vi "SS GUI Measurement setup.vi"(9 "SS measurement":T1={"Signal frequencies (Hz)"=[1000.0], "Signal amplitudes (V)"=[0.707], "Sampling frequencies (Hz)"=[10000000.0], "Record lengths (multiples of periods)"=[10000.0], "Calculate results"=FALSE, "Algorithm"="TWM-WFFT", "TWM data directories"=[], "TWM data directories relative"=[], "Settle down after AC source change (s)"=1.0, "PJVS frequencies (Hz)"=[1000.0], "PJVS reference voltages array of vector cluster"=[{"PJVS reference voltages vector"=[]}], "Requested PJVS steps"=[20], "Measure CE"=FALSE, "Measure CE before"=FALSE, "Measure CE after"=FALSE, "Single point CE measurement"=FALSE, "original CE template path"=path "", "new CE template path before SS"=path "", "new CE template path before SS relative"=path "", "new CE template path after SS"=path "", "new CE template path after SS relative"=path "", "original CE fit path"=path "", "new CE fit path before SS"=path "", "new CE fit path before SS relative"=path "", "new CE fit path after SS"=path "", "new CE fit path after SS relative"=path "", "Measure digitizer gain"=FALSE, "Measure digitizer gain before"=FALSE, "Measure digitizer gain after"=FALSE, "Digitizer gain"=0.0, "Data folder"=path "", "FR fit path"=path "", "new FR fit path relative"=path "", "Rs"=0, "Re"=0, "SS measurement info files"=[]} {"PJVS reference voltages array of vector cluster"."PJVS reference voltages vector" format="%#_3p"; "PJVS frequencies (Hz)" format="%#_3p"; "Record lengths (multiples of periods)" format="%#_3p"; "Sampling frequencies (Hz)" format="%#_3p"; "Signal amplitudes (V)" format="%#_3p"; "Signal frequencies (Hz)" format="%#_3p"}) -> (3 "SS measurement out":T1={"Signal frequencies (Hz)"=[1000.0], "Signal amplitudes (V)"=[0.707], "Sampling frequencies (Hz)"=[10000000.0], "Record lengths (multiples of periods)"=[10000.0], "Calculate results"=FALSE, "Algorithm"="TWM-WFFT", "TWM data directories"=[], "TWM data directories relative"=[], "Settle down after AC source change (s)"=1.0, "PJVS frequencies (Hz)"=[1000.0], "PJVS reference voltages array of vector cluster"=[{"PJVS reference voltages vector"=[]}], "Requested PJVS steps"=[20], "Measure CE"=FALSE, "Measure CE before"=FALSE, "Measure CE after"=FALSE, "Single point CE measurement"=FALSE, "original CE template path"=path "", "new CE template path before SS"=path "", "new CE template path before SS relative"=path "", "new CE template path after SS"=path "", "new CE template path after SS relative"=path "", "original CE fit path"=path "", "new CE fit path before SS"=path "", "new CE fit path before SS relative"=path "", "new CE fit path after SS"=path "", "new CE fit path after SS relative"=path "", "Measure digitizer gain"=FALSE, "Measure digitizer gain before"=FALSE, "Measure digitizer gain after"=FALSE, "Digitizer gain"=0.0, "Data folder"=path "", "FR fit path"=path "", "new FR fit path relative"=path "", "Rs"=0, "Re"=0, "SS measurement info files"=[]} {"PJVS reference voltages array of vector cluster"."PJVS reference voltages vector" format="%#_3p"; "PJVS frequencies (Hz)" format="%#_3p"; "Record lengths (multiples of periods)" format="%#_3p"; "Sampling frequencies (Hz)" format="%#_3p"; "Signal amplitudes (V)" format="%#_3p"; "Signal frequencies (Hz)" format="%#_3p"})   [LabVIEW 2020]
uses:
  SS Measurement/Type definitions/SS measurement.ctl
  <vilib>/Utility/error.llb/Error Cluster From Error Code.vi
  <vilib>/ErrorRing/Error Ring.xnode
  external libraries/varilib/varilib.lvlib
panel:
  in  "TabCEmeas":enum32{"Measure CE", "Without CE meas."}(tab)
  in  "Measure CE before":bool caption="before"
  in  "Measure CE after":bool caption="after"
  in  "RadioCEmeastype":enum32{"single point", "template"}(radio) caption="Method:"
  in  "orignal CE template path":path caption="CE template path:"
  in  "original CE fit path":path caption="Use file with CE fit:"
  in  "Re":i32 min=0 step=1
  in  "Rs":i32 min=0 step=1
  out "PJVS triangles error":string="!"
  out "PJVS triangles in record":dbl
  out "No of samples":dbl format="%#_6p"
  out "Sampling time (s)":dbl
  in  "original FR fit path":path caption="FR fit path:"
  out "DG error":string="!"
  in  "RadioGain":enum32{"DGmeasure", "DGvalue"}(radio)
  in  "Measure gain after":bool caption="after"
  in  "Measure gain before":bool caption="before"
  in  "Digitizer gain":dbl=1.0 min=1e-07 max=10000000000.0 format="%_7g"
  out "Is coherent":string="!"
  out "CE error":string="!"
  in  "Data folder":path caption="Save data to folder:"
  in  "Requested PJVS steps":u32
  out "Requested PJVS steps out":u32[](array[numeric])
  in  "PJVS frequency (Hz)":dbl
  out "PJVS frequencies (Hz) out":dbl[](array[numeric])
  in  "Record length (multiple of period)":dbl
  in  "Signal frequency (Hz)":dbl format="%#_7p"
  in  "Calculate results":bool
  in  "Algorithm":string
  out "Signal amplitudes (V) out":dbl[](array[numeric])
  out "Record lengths (multiples of period)":dbl[](array[numeric])
  out "Sampling frequencies (Hz) out":dbl[](array[numeric])
  out "Signal frequencies out (Hz)":dbl[](array[numeric]) caption="List of measurement frequencies" format="%#_7p"
  in  "Settle down after AC\nsource change (s)":dbl=1.0 format="%#_13g"
  in  "Sampling frequency (Hz)":dbl=10000000.0 format="%#_13p"
  in  "Signal amplitude (V)":dbl=1.0 format="%#_13g"
  in  "show connections":bool
  out "gui_elements":refnum<vi>[](array[refnum])
  in  "save_and_quit":bool
  in  "cancel":bool
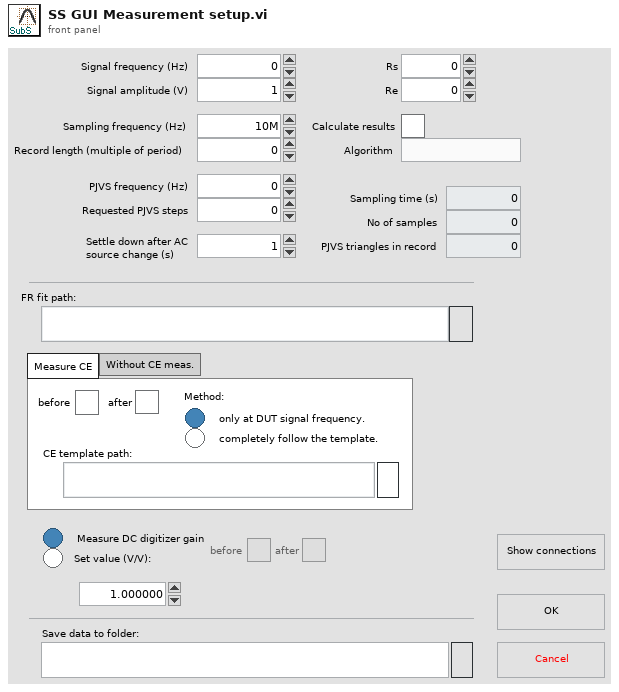
[diagram p1: front panel]
types:
  T1 = typedef "SS measurement.ctl" = cluster{"Signal frequencies (Hz)":dbl[], "Signal amplitudes (V)":dbl[], "Sampling frequencies (Hz)":dbl[], "Record lengths (multiples of periods)":dbl[], "Calculate results":bool, "Algorithm":string, "TWM data directories":path[], "TWM data directories relative":path[], "Settle down after AC source change (s)":dbl, "PJVS frequencies (Hz)":dbl[], "PJVS reference voltages array of vector cluster":cluster{"PJVS reference voltages vector":dbl[]}[], "Requested PJVS steps":u32[], "Measure CE":bool, "Measure CE before":bool, "Measure CE after":bool, "Single point CE measurement":bool, "original CE template path":path, "new CE template path before SS":path, "new CE template path before SS relative":path, "new CE template path after SS":path, "new CE template path after SS relative":path, "original CE fit path":path, "new CE fit path before SS":path, "new CE fit path before SS relative":path, "new CE fit path after SS":path, "new CE fit path after SS relative":path, "Measure digitizer gain":bool, "Measure digitizer gain before":bool, "Measure digitizer gain after":bool, "Digitizer gain":dbl, "Data folder":path, "FR fit path":path, "new FR fit path relative":path, "Rs":i32, "Re":i32, "SS measurement info files":path[]}
  T2 = enum32{"Bad", "Idle", "Run top level", "Running"}
  T3 = cluster{"PJVS reference voltages vector":dbl[]}[]
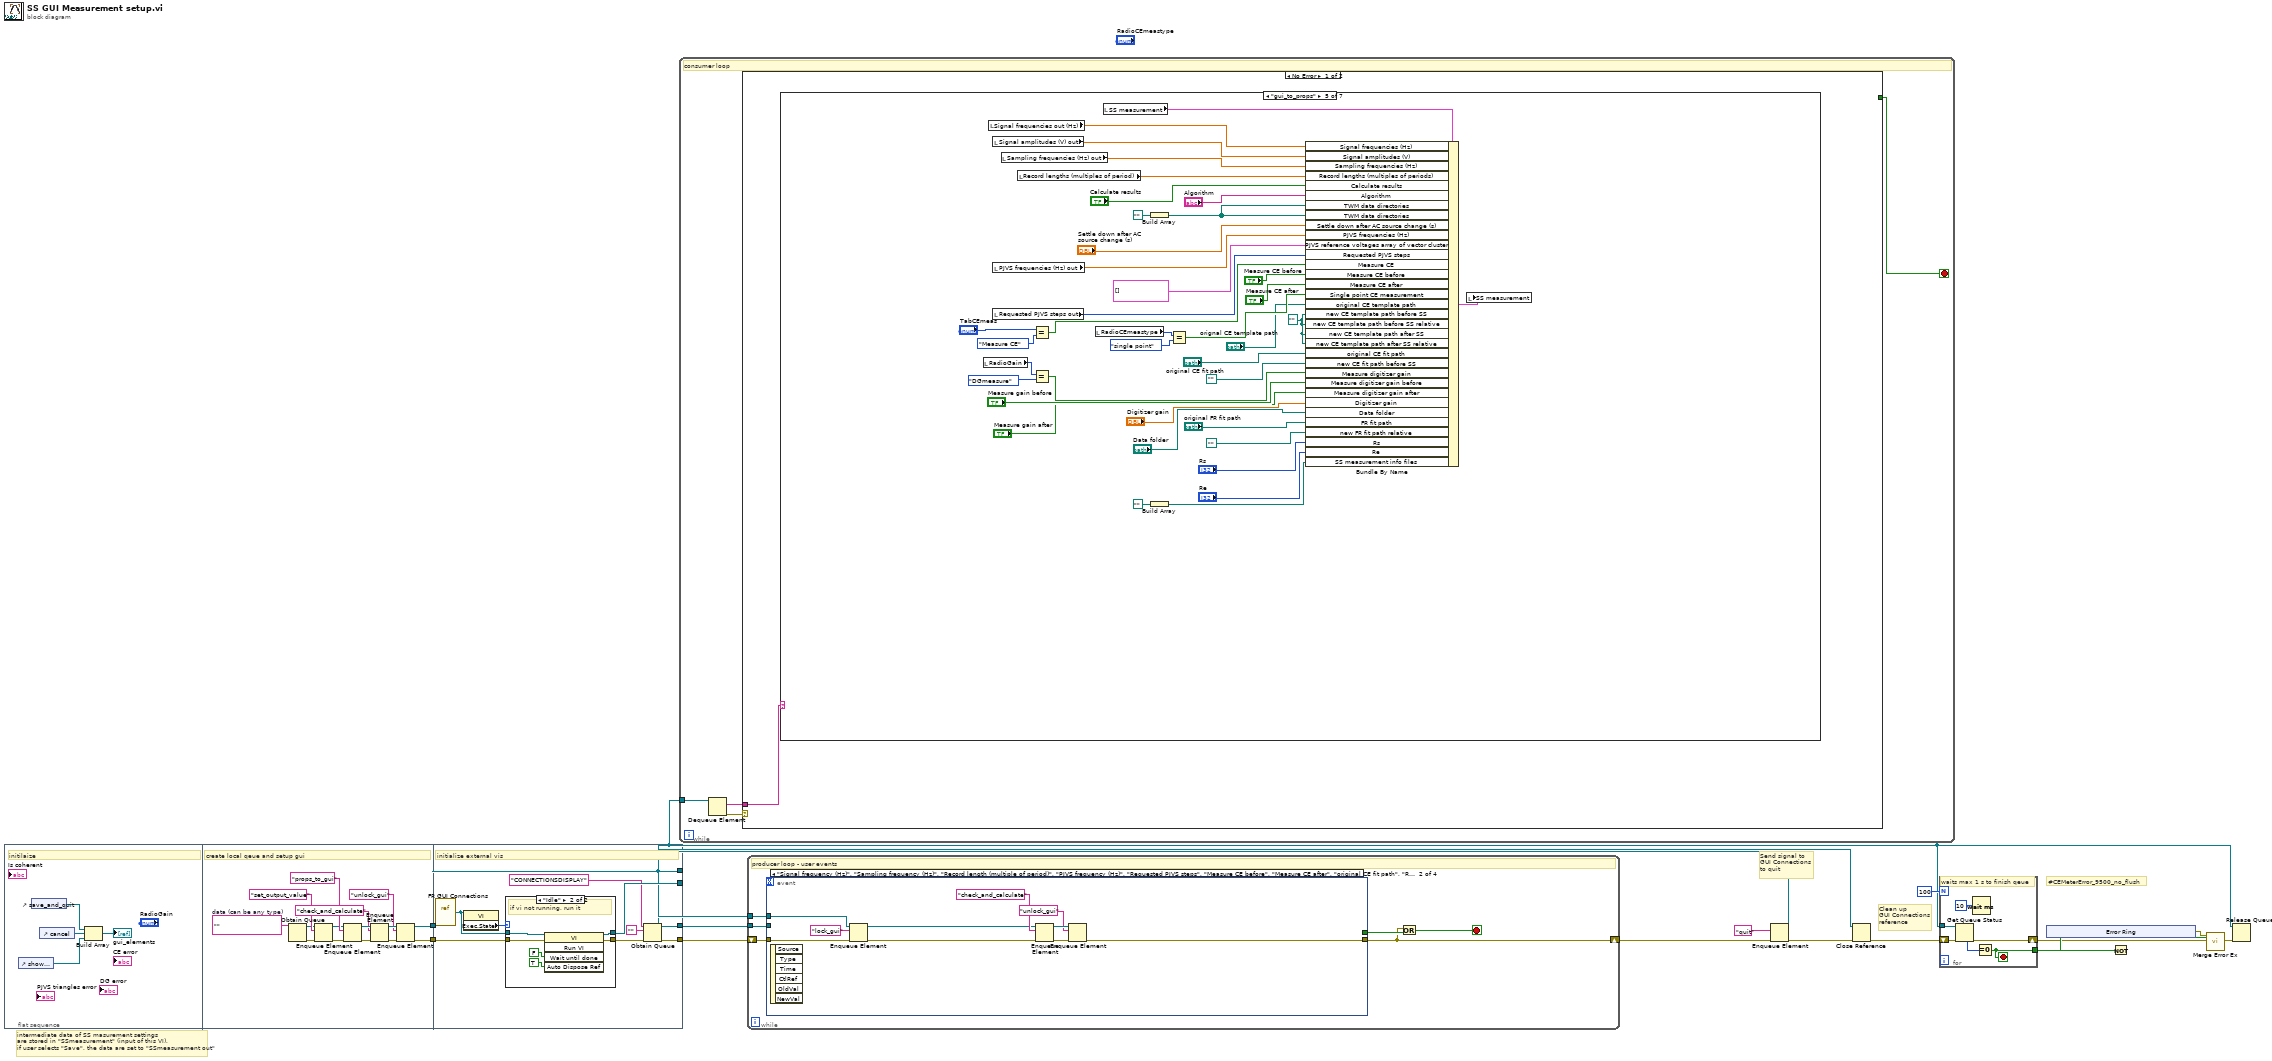
[diagram p0: block diagram]
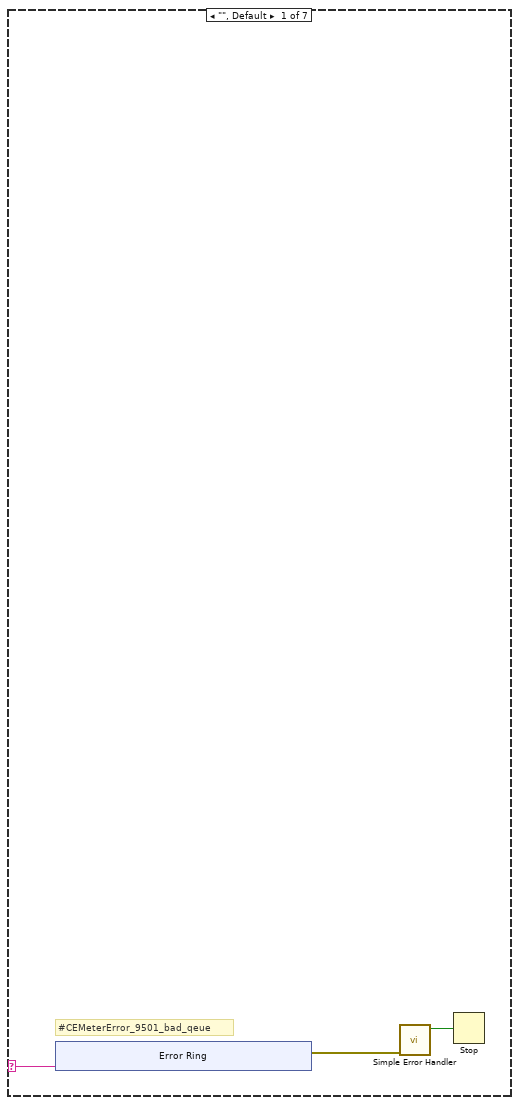
[diagram p3: hidden frame]
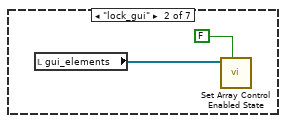
[diagram p4: hidden frame]
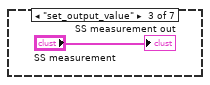
[diagram p5: hidden frame]
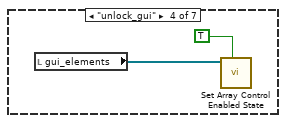
[diagram p6: hidden frame]
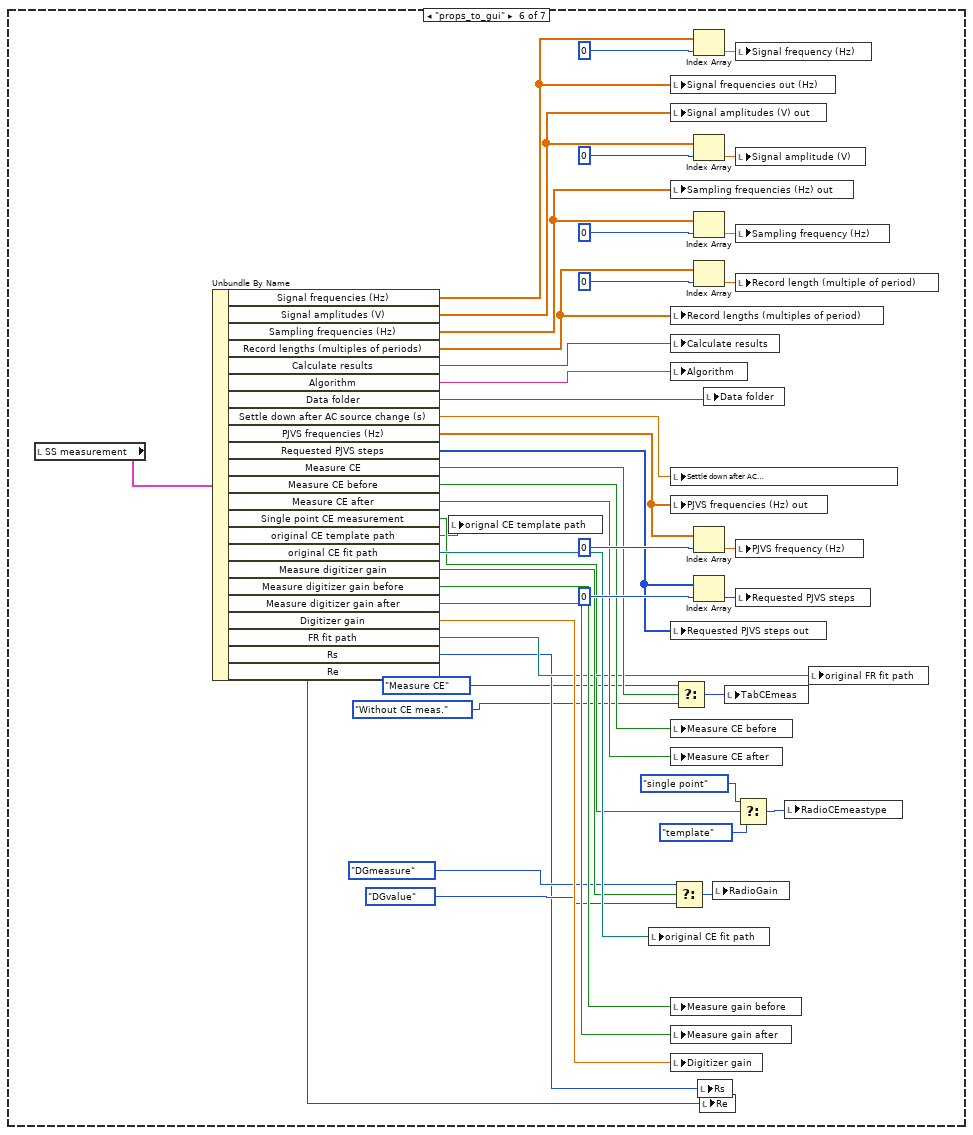
[diagram p7: hidden frame]
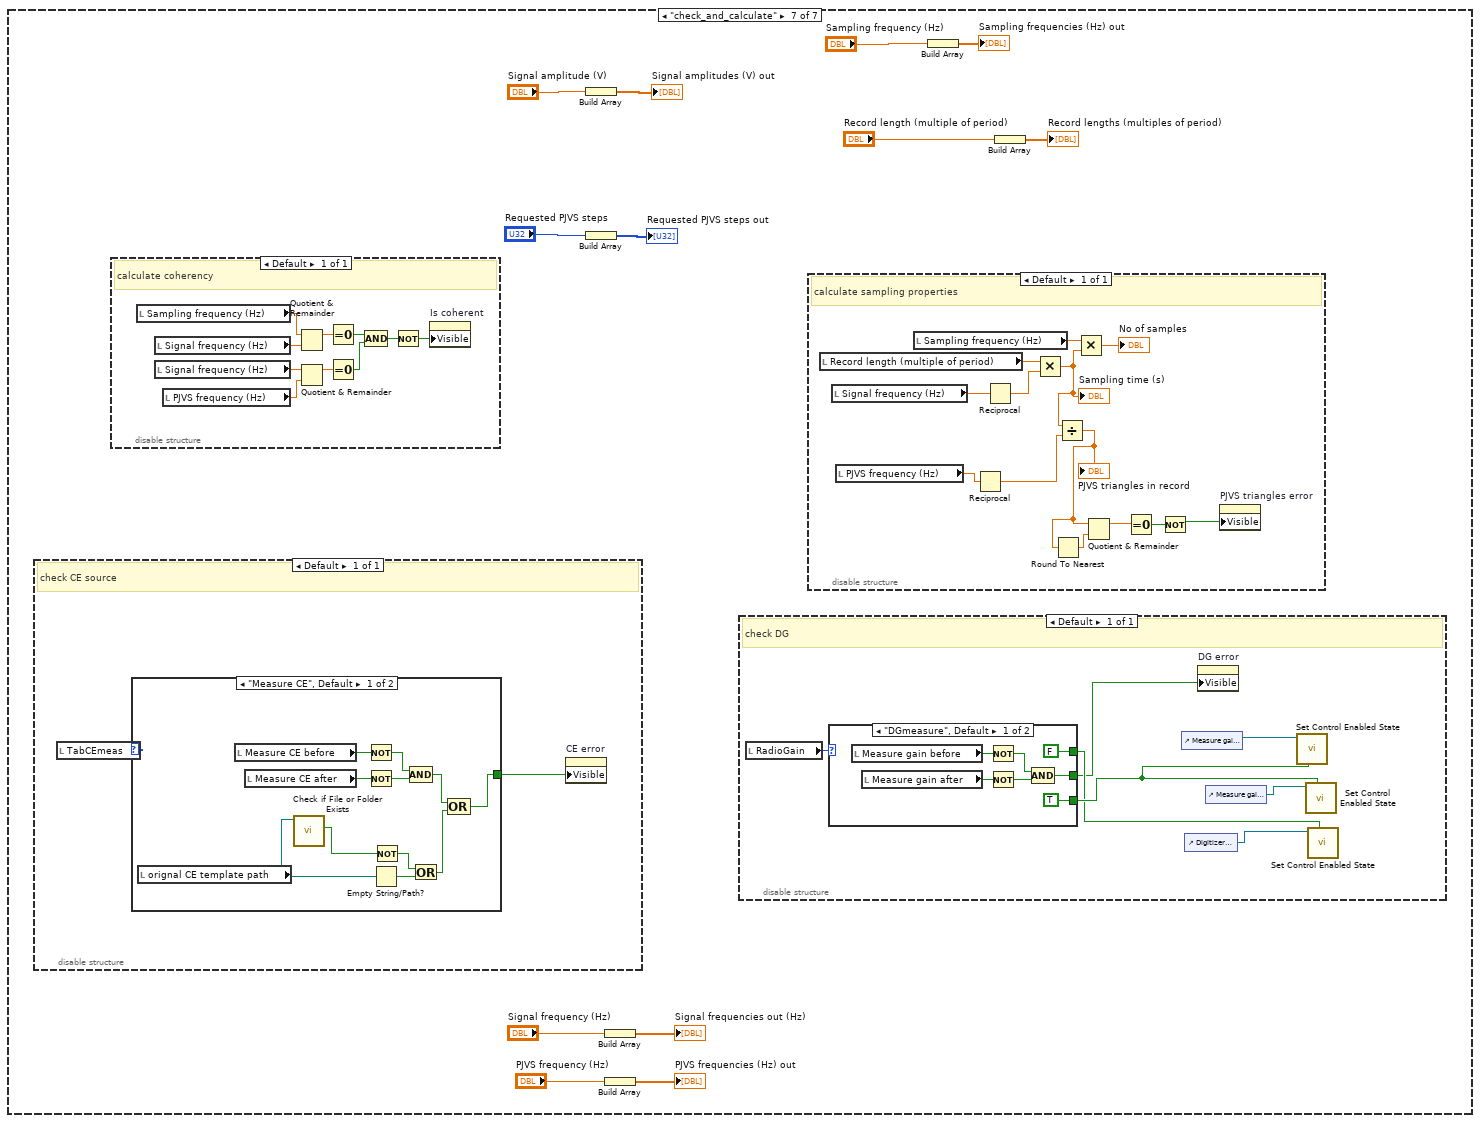
[diagram p8: hidden frame]
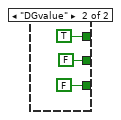
[diagram p9: hidden frame]
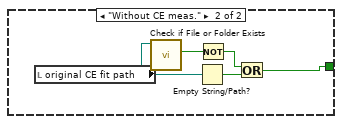
[diagram p10: hidden frame]
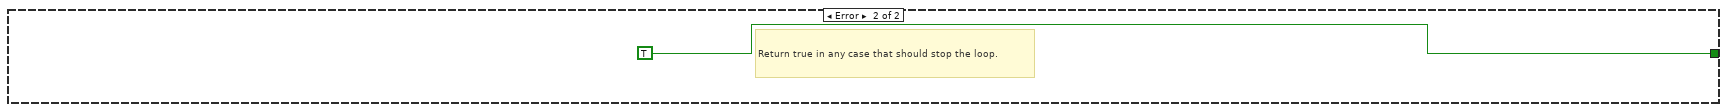
[diagram p11: hidden frame]
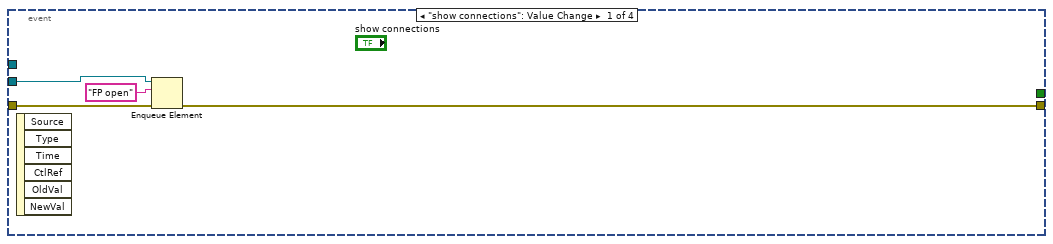
[diagram p12: hidden frame]
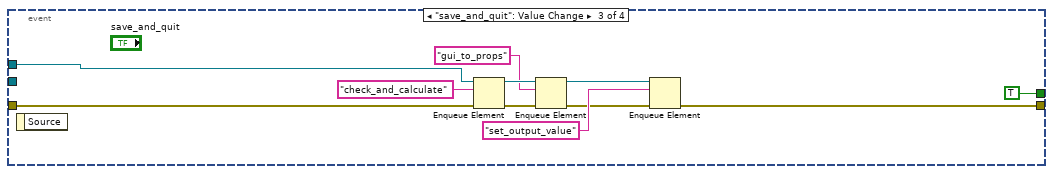
[diagram p13: hidden frame]
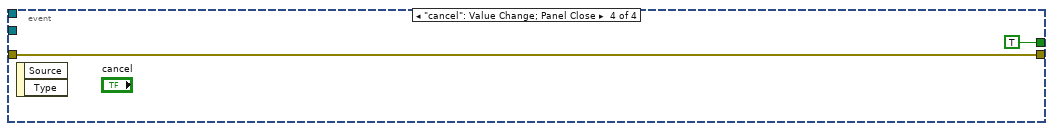
[diagram p14: hidden frame]
diagram:
  # "intermediate data of SS masurement settings\nare stored in \"SSmeasurement\" (input of this VI),\nif user selects \"Save\", the data are set to \"SSmeasurement out\""
  # "Send signal to\nGUI Connections\nto quit"
  # "Clean up\nGUI Connections\nreference"
  # "#CEMeterError_9500_no_flush"
  n1 = flat-sequence {
    tunnel: [w25] -> w9
    tunnel: [w24] -> w1
    tunnel: [w41] -> w10
    tunnel: [w45] -> w4
    tunnel: w9 -> [w44]
    tunnel: [w42] -> w3
    tunnel: [w43] -> w6
    tunnel: w1 -> [w45]
    frame #0 {
      # "initilaize"
      n2 = control-ref of="show connections"() -> (w17:refnum<vi>)
      n3 = control-ref of="save_and_quit"() -> (w20:refnum<vi>)
      n4 = control-ref of="cancel"() -> (w19:refnum<vi>)
      n5 = Build Array(w20, w19, w17) -> (→"gui_elements":refnum<vi>[])
    }
    frame #1 {
      w34 = ""  # data (can be any type)
      # "create local qeue and setup gui"
      n6 = Obtain Queue(element data type=w34) -> (queue out=w27:refnum<queue>, error out=w26:errorcluster)  [unwired: 4 in, 1 out]
      n7 = Enqueue Element(queue=w27, element="set_output_value", error in (no error)=w26) -> (queue out=w29:refnum<queue>, error out=w28:errorcluster)  [unwired: 1 in, 1 out]
      n8 = Enqueue Element(queue=w29, element="props_to_gui", error in (no error)=w28) -> (queue out=w32:refnum<queue>, error out=w33:errorcluster)  [unwired: 1 in, 1 out]
      n9 = Enqueue Element(queue=w32, element="check_and_calculate", error in (no error)=w33) -> (queue out=w23:refnum<queue>, error out=w22:errorcluster)  [unwired: 1 in, 1 out]
      n10 = Enqueue Element(queue=w23, element="unlock_gui", error in (no error)=w22) -> (queue out=w24:refnum<queue>, error out=w25:errorcluster)  [unwired: 1 in, 1 out]
    }
    frame #2 {
      # "initialize external vis"
      n11 = vi-ref "FR GUI Connections.vi"() -> (w39:refnum<vi>)
      n12 = property class="VI"(reference=w39) -> ("Exec.State"=w40:T2)  [unwired: 1 in, 2 out]
      n13 = case shown="\"Idle\"" w40 {
        tunnel: [w46 w53] -> w36
        tunnel: w44 -> [w46 w50]
        tunnel: [w47 w49] -> w43
        tunnel: w39 -> [w47 w48]
        frame "Bad", Default {
        }
        frame "Idle" {
          # "if vi not running, run it"
          n14 = invoke class="VI" method="Run VI"(reference=w48, error in=w50, "Wait until done"=FALSE ("Wait Until Done"), "Auto Dispose Ref"=TRUE ("Wait Until Done")) -> (reference out=w49:refnum<vi>, error out=w53:errorcluster)  [unwired: 1 in, 3 out]
        }
      }
      n15 = Obtain Queue(name (unnamed)="CONNECTIONSDISPLAY", element data type="", error in (no error)=w36) -> (queue out=w42:refnum<queue>, error out=w41:errorcluster)  [unwired: 2 in, 1 out]
    }
  }
  n16 = while {
    tunnel: w4 -> [w57]
    stop <- w54 stop-if-true
    # "consumer loop"
    n17 = Dequeue Element(queue=w57) -> (element=w55:string, error out=w56:errorcluster)  [unwired: 2 in, 2 out]
    n18 = case shown="No Error" w56 {
      tunnel: w55 -> [w58 _]
      tunnel: [_ TRUE] -> w54
      frame No Error {
        n19 = case shown="\"gui_to_props\"" w58 {
          selector: w58 -> [w59 _ _ _ _ _ _]
          frame "", Default {
            # "#CEMeterError_9501_bad_qeue"
            n20 = xnode "Error Ring"("parameter 0"=w59) -> ("error out"=w61:errorcluster)
            n21 = call <vilib>:"Simple Error Handler.vi"("error in (no error)"=w61) -> ("error?"=w60:bool)  [unwired: 4 in, 4 out]
            n22 = Stop(stop? (T)=w60) -> ()
          }
          frame "lock_gui" {
            n23 = local read "gui_elements"() -> (w70:refnum<vi>[])
            n24 = call "Set Array Control Enabled State.vi"("enabled (T)"=FALSE, "reference array in"=w70) -> ()  [unwired: 8 in, 2 out]
          }
          frame "set_output_value" {
            "SS measurement out" <- "SS measurement"
          }
          frame "unlock_gui" {
            n25 = local read "gui_elements"() -> (w73:refnum<vi>[])
            n26 = call "Set Array Control Enabled State.vi"("enabled (T)"=TRUE, "reference array in"=w73) -> ()  [unwired: 8 in, 2 out]
          }
          frame "gui_to_props" {
            w80 = path ""
            n27 = local read "RadioGain"() -> (w94:enum32{"DGmeasure", "DGvalue"})
            n28 = local read "Signal frequencies out (Hz)"() -> (w104:dbl[])
            n29 = local read "Signal amplitudes (V) out"() -> (w110:dbl[])
            n30 = local read "PJVS frequencies (Hz) out"() -> (w103:dbl[])
            n31 = local read "Requested PJVS steps out"() -> (w102:u32[])
            n32 = local read "Sampling frequencies (Hz) out"() -> (w109:dbl[])
            n33 = local read "Record lengths (multiples of period)"() -> (w108:dbl[])
            n34 = Equal?(x="TabCEmeas", y=enum32{"Measure CE", "Without CE meas."}."Measure CE" ("TabCEmeas")) -> (x = y?=w95:bool)
            n35 = Equal?(x=w94, y=enum32{"DGmeasure", "DGvalue"}."DGmeasure" ("RadioGain")) -> (x = y?=w93:bool)
            n36 = local read "RadioCEmeastype"() -> (w79:enum32{"single point", "template"})
            n37 = local read "SS measurement"() -> (w111:T1)
            n38 = Build Array(path "") -> (w87:path[])
            n39 = Build Array(path "") -> (w82:path[])
            n40 = Equal?(x=w79, y=enum32{"single point", "template"}."single point" ("RadioCEmeastype")) -> (x = y?=w77:bool)
            n41 = Bundle By Name(cluster=w111, "Signal frequencies (Hz)"=w104, "Signal amplitudes (V)"=w110, "Sampling frequencies (Hz)"=w109, "Record lengths (multiples of periods)"=w108, "Calculate results"="Calculate results", "Algorithm"="Algorithm", "TWM data directories"=w87, "TWM data directories"=w87, "Settle down after AC source change (s)"="Settle down after AC\nsource change (s)", "PJVS frequencies (Hz)"=w103, "PJVS reference voltages array of vector cluster"=T3 [], "Requested PJVS steps"=w102, "Measure CE"=w95, "Measure CE before"="Measure CE before", "Measure CE after"="Measure CE after", "Single point CE measurement"=w77, "original CE template path"="orignal CE template path", "new CE template path before SS"=w80, "new CE template path before SS relative"=w80, "new CE template path after SS"=w80, "new CE template path after SS relative"=w80, "original CE fit path"="original CE fit path", "new CE fit path before SS"=path "", "Measure digitizer gain"=w93, "Measure digitizer gain before"="Measure gain before", "Measure digitizer gain after"="Measure gain after", "Digitizer gain"="Digitizer gain", "Data folder"="Data folder", "FR fit path"="original FR fit path", "new FR fit path relative"=path "", "Rs"="Rs", "Re"="Re", "SS measurement info files"=w82) -> (w112:T1)
            n42 = local write "SS measurement"(w112) -> ()
          }
          frame "props_to_gui" {
            n43 = local read "SS measurement"() -> (w157:T1)
            n44 = Unbundle By Name(w157) -> ("Signal frequencies (Hz)"=w150:dbl[], "Signal amplitudes (V)"=w149:dbl[], "Sampling frequencies (Hz)"=w148:dbl[], "Record lengths (multiples of periods)"=w146:dbl[], "Calculate results"=w144:bool, "Algorithm"=w143:string, "Data folder"=w124:path, "Settle down after AC source change (s)"=w142:dbl, "PJVS frequencies (Hz)"=w137:dbl[], "Requested PJVS steps"=w130:u32[], "Measure CE"=w129:bool, "Measure CE before"=w134:bool, "Measure CE after"=w135:bool, "Single point CE measurement"=w120:bool, "original CE template path"=w113:path, "original CE fit path"=w136:path, "Measure digitizer gain"=w128:bool, "Measure digitizer gain before"=w133:bool, "Measure digitizer gain after"=w132:bool, "Digitizer gain"=w131:dbl, "FR fit path"=w123:path, "Rs"=w122:i32, "Re"=w121:i32)
            n45 = local write "orignal CE template path"(w113) -> ()
            n46 = local write "original CE fit path"(w136) -> ()
            n47 = local write "Signal frequencies out (Hz)"(w150) -> ()
            n48 = local write "Signal amplitudes (V) out"(w149) -> ()
            n49 = local write "Sampling frequencies (Hz) out"(w148) -> ()
            n50 = local write "Record lengths (multiples of period)"(w146) -> ()
            n51 = local write "Calculate results"(w144) -> ()
            n52 = local write "Algorithm"(w143) -> ()
            n53 = local write "Settle down after AC\nsource change (s)"(w142) -> ()
            n54 = local write "PJVS frequencies (Hz) out"(w137) -> ()
            n55 = local write "Requested PJVS steps out"(w130) -> ()
            n56 = local write "Measure CE before"(w134) -> ()
            n57 = local write "Measure CE after"(w135) -> ()
            n58 = local write "Measure gain before"(w133) -> ()
            n59 = local write "Measure gain after"(w132) -> ()
            n60 = local write "Digitizer gain"(w131) -> ()
            n61 = Select(t=enum32{"DGmeasure", "DGvalue"}."DGmeasure" ("RadioGain"), s=w128, f=enum32{"DGmeasure", "DGvalue"}."DGvalue" ("RadioGain")) -> (s? t:f=w125:enum32{"DGmeasure", "DGvalue"})
            n62 = Select(t=enum32{"Measure CE", "Without CE meas."}."Measure CE" ("TabCEmeas"), s=w129, f=enum32{"Measure CE", "Without CE meas."}."Without CE meas." ("TabCEmeas")) -> (s? t:f=w115:enum32{"Measure CE", "Without CE meas."})
            n63 = Index Array(array=w150, index=0) -> (element=w153:dbl)
            n64 = Index Array(array=w149, index=0) -> (element=w156:dbl)
            n65 = Index Array(array=w148, index=0) -> (element=w151:dbl)
            n66 = Index Array(array=w146, index=0) -> (element=w145:dbl)
            n67 = Index Array(array=w137, index=0) -> (element=w138:dbl)
            n68 = Index Array(array=w130, index=0) -> (element=w139:u32)
            n69 = local write "Rs"(w122) -> ()
            n70 = local write "Re"(w121) -> ()
            n71 = local write "Data folder"(w124) -> ()
            n72 = local write "RadioGain"(w125) -> ()
            n73 = local write "TabCEmeas"(w115) -> ()
            n74 = local write "Signal frequency (Hz)"(w153) -> ()
            n75 = local write "Signal amplitude (V)"(w156) -> ()
            n76 = local write "Sampling frequency (Hz)"(w151) -> ()
            n77 = local write "Record length (multiple of period)"(w145) -> ()
            n78 = local write "PJVS frequency (Hz)"(w138) -> ()
            n79 = local write "Requested PJVS steps"(w139) -> ()
            n80 = Select(t=enum32{"single point", "template"}."single point" ("CE measurement type"), s=w120, f=enum32{"single point", "template"}."template" ("CE measurement type")) -> (s? t:f=w117:enum32{"single point", "template"})
            n81 = local write "RadioCEmeastype"(w117) -> ()
            n82 = local write "original FR fit path"(w123) -> ()
          }
          frame "check_and_calculate" {
            n83 = disable-structure shown="Default" {
              frame Enabled {
                # "check CE source"
                n84 = local read "TabCEmeas"() -> (w210:enum32{"Measure CE", "Without CE meas."})
                n85 = case shown="\"Measure CE\", Default" w210 {
                  tunnel: [w213 w223] -> w211
                  frame "Measure CE", Default {
                    n86 = local read "orignal CE template path"() -> (w216:path)
                    n87 = local read "Measure CE before"() -> (w222:bool)
                    n88 = local read "Measure CE after"() -> (w219:bool)
                    n89 = call <vilib>:"Check if File or Folder Exists.vi"("path"=w216) -> ("file or folder exists?"=w215:bool)  [unwired: 8 in, 2 out]
                    n90 = Not(x=w222) -> (.not. x?=w221:bool)
                    n91 = Not(x=w219) -> (.not. x?=w220:bool)
                    n92 = Empty String/Path?(string/path=w216) -> (empty?=w218:bool)
                    n93 = Not(x=w215) -> (.not. x?=w217:bool)
                    n94 = Compound Arithmetic op=AND(w221, w220) -> (w214:bool)
                    n95 = Or(x=w217, y=w218) -> (x .or. y?=w212:bool)
                    n96 = Compound Arithmetic op=OR(w214, w212) -> (w213:bool)
                  }
                  frame "Without CE meas." {
                    n97 = local read "original CE fit path"() -> (w225:path)
                    n98 = call <vilib>:"Check if File or Folder Exists.vi"("path"=w225) -> ("file or folder exists?"=w224:bool)  [unwired: 8 in, 2 out]
                    n99 = Empty String/Path?(string/path=w225) -> (empty?=w226:bool)
                    n100 = Not(x=w224) -> (.not. x?=w227:bool)
                    n101 = Or(x=w227, y=w226) -> (x .or. y?=w223:bool)
                  }
                }
                n102 = property on="CE error" class="Str"("Visible"=w211) -> ()  [unwired: 2 in, 2 out]
              }
            }
            n103 = disable-structure shown="Default" {
              frame Enabled {
                # "calculate coherency"
                n104 = local read "Sampling frequency (Hz)"() -> (w209:dbl)
                n105 = local read "Signal frequency (Hz)"() -> (w208:dbl)
                n106 = local read "Signal frequency (Hz)"() -> (w201:dbl)
                n107 = local read "PJVS frequency (Hz)"() -> (w200:dbl)
                n108 = Quotient & Remainder(x=w209, y=w208) -> (x-y*floor(x/y)=w207:dbl)  [unwired: 1 out]
                n109 = Quotient & Remainder(x=w201, y=w200) -> (x-y*floor(x/y)=w205:dbl)  [unwired: 1 out]
                n110 = Equal To 0?(x=w207) -> (x = 0?=w206:bool)
                n111 = Equal To 0?(x=w205) -> (x = 0?=w204:bool)
                n112 = Compound Arithmetic op=AND(w206, w204) -> (w203:bool)
                n113 = Not(x=w203) -> (.not. x?=w202:bool)
                n114 = property on="Is coherent" class="Str"("Visible"=w202) -> ()  [unwired: 2 in, 2 out]
              }
            }
            n115 = Build Array("Signal amplitude (V)") -> (→"Signal amplitudes (V) out":dbl[])
            n116 = Build Array("Requested PJVS steps") -> (→"Requested PJVS steps out":u32[])
            n117 = Build Array("Signal frequency (Hz)") -> (→"Signal frequencies out (Hz)":dbl[])
            n118 = Build Array("PJVS frequency (Hz)") -> (→"PJVS frequencies (Hz) out":dbl[])
            n119 = disable-structure shown="Default" {
              frame Enabled {
                # "check DG"
                n120 = local read "RadioGain"() -> (w189:enum32{"DGmeasure", "DGvalue"})
                n121 = case shown="\"DGmeasure\", Default" w189 {
                  tunnel: [w192 FALSE] -> w183
                  tunnel: [TRUE ("enabled (T)") FALSE ("enabled (T)")] -> w185
                  tunnel: [FALSE ("enabled (T)") TRUE ("enabled (T)")] -> w184
                  frame "DGmeasure", Default {
                    n122 = local read "Measure gain before"() -> (w196:bool)
                    n123 = local read "Measure gain after"() -> (w193:bool)
                    n124 = Not(x=w196) -> (.not. x?=w195:bool)
                    n125 = Not(x=w193) -> (.not. x?=w194:bool)
                    n126 = Compound Arithmetic op=AND(w195, w194) -> (w192:bool)
                  }
                  frame "DGvalue" {
                  }
                }
                n127 = control-ref of="Measure gain before"() -> (w188:refnum<vi>)
                n128 = control-ref of="Digitizer gain"() -> (w186:refnum<vi>)
                n129 = property on="DG error" class="Str"("Visible"=w183) -> ()  [unwired: 2 in, 2 out]
                n130 = control-ref of="Measure gain after"() -> (w187:refnum<vi>)
                n131 = call "Set Control Enabled State.vi"("enabled (T)"=w185, "reference in"=w188) -> ()  [unwired: 8 in, 2 out]
                n132 = call "Set Control Enabled State.vi"("enabled (T)"=w185, "reference in"=w187) -> ()  [unwired: 8 in, 2 out]
                n133 = call "Set Control Enabled State.vi"("enabled (T)"=w184, "reference in"=w186) -> ()  [unwired: 8 in, 2 out]
              }
            }
            n134 = disable-structure shown="Default" {
              frame Enabled {
                # "calculate sampling properties"
                n135 = local read "Record length (multiple of period)"() -> (w180:dbl)
                n136 = local read "Signal frequency (Hz)"() -> (w182:dbl)
                n137 = local read "PJVS frequency (Hz)"() -> (w177:dbl)
                n138 = local read "Sampling frequency (Hz)"() -> (w179:dbl)
                n139 = Reciprocal(x=w177) -> (1/x=w176:dbl)
                n140 = Reciprocal(x=w182) -> (1/x=w181:dbl)
                n141 = Multiply(x=w180, y=w181) -> (x*y=w175:dbl)
                "Sampling time (s)" <- w175
                n142 = Divide(x=w175, y=w176) -> (x/y=w173:dbl)
                "PJVS triangles in record" <- w173
                n143 = Round To Nearest(number=w173) -> (nearest integer value=w174:dbl)
                n144 = Multiply(x=w179, y=w175) -> (x*y=→"No of samples":dbl)
                n145 = Quotient & Remainder(x=w173, y=w174) -> (x-y*floor(x/y)=w172:dbl)  [unwired: 1 out]
                n146 = Equal To 0?(x=w172) -> (x = 0?=w171:bool)
                n147 = Not(x=w171) -> (.not. x?=w170:bool)
                n148 = property on="PJVS triangles error" class="Str"("Visible"=w170) -> ()  [unwired: 2 in, 2 out]
              }
            }
            n149 = Build Array("Sampling frequency (Hz)") -> (→"Sampling frequencies (Hz) out":dbl[])
            n150 = Build Array("Record length (multiple of period)") -> (→"Record lengths (multiples of period)":dbl[])
          }
        }
      }
      frame Error {
        # "Return true in any case that should stop the loop."
      }
    }
  }
  n151 = while {
    shift-right: [w230] -> w5
    shift-left: w10 -> [w233]
    tunnel: w4 -> [w234]
    tunnel: w3 -> [w229]
    stop <- w231 stop-if-true
    # "producer loop - user events"
    n152 = event shown="[1] \"Signal frequency (Hz)\", \"Sampling frequency (Hz)\", \"Record length (multiple of period)\", \"PJVS frequency (Hz)\", \"Requested PJVS steps\", \"Measure CE before\", \"Measure CE after\", \"original CE fit path\", \"RadioGain\", \"Measure gain before\", \"Measure gain after\", \"TabCEmeas\": Value Change" {
      selector: _ -> [_ _ _ _]
      dyn-events: _ -> [_ _ _ _]
      timeout: _ -> [_ _ _ _]
      tunnel: w234 -> [_ w247 w258 _]
      tunnel: w233 -> [w237 w240 w257 w260]
      tunnel: [w236 w239 w256 w260] -> w230
      tunnel: [_ _ TRUE ("cancel") TRUE ("cancel")] -> w232
      tunnel: w229 -> [w235 _ _ _]
      event "show connections": Value Change {
        n153 = event-data() -> ()  [unwired: 1 in, 6 out]
        n154 = Enqueue Element(queue=w235, element="FP open", error in (no error)=w237) -> (error out=w236:errorcluster)  [unwired: 1 in, 2 out]
      }
      event "Signal frequency (Hz)", "Sampling frequency (Hz)", "Record length (multiple of period)", "PJVS frequency (Hz)", "Requested PJVS steps", "Measure CE before", "Measure CE after", "original CE fit path", "RadioGain", "Measure gain before", "Measure gain after", "TabCEmeas": Value Change {
        n155 = event-data() -> ()  [unwired: 1 in, 6 out]
        n156 = Enqueue Element(queue=w247, element="lock_gui", error in (no error)=w240) -> (queue out=w246:refnum<queue>, error out=w241:errorcluster)  [unwired: 1 in, 1 out]
        n157 = Enqueue Element(queue=w246, element="check_and_calculate", error in (no error)=w241) -> (queue out=w245:refnum<queue>, error out=w242:errorcluster)  [unwired: 1 in, 1 out]
        n158 = Enqueue Element(queue=w245, element="unlock_gui", error in (no error)=w242) -> (error out=w239:errorcluster)  [unwired: 1 in, 2 out]
      }
      event "save_and_quit": Value Change {
        n159 = event-data() -> ()  [unwired: 1 in, 1 out]
        n160 = Enqueue Element(queue=w258, element="check_and_calculate", error in (no error)=w257) -> (queue out=w253:refnum<queue>, error out=w254:errorcluster)  [unwired: 1 in, 1 out]
        n161 = Enqueue Element(queue=w253, element="gui_to_props", error in (no error)=w254) -> (queue out=w252:refnum<queue>, error out=w251:errorcluster)  [unwired: 1 in, 1 out]
        n162 = Enqueue Element(queue=w252, element="set_output_value", error in (no error)=w251) -> (error out=w256:errorcluster)  [unwired: 1 in, 2 out]
      }
      event "cancel": Value Change; Panel Close {
        n163 = event-data() -> ()  [unwired: 1 in, 2 out]
      }
    }
    n164 = Or(x=w230, y=w232) -> (x .or. y?=w231:bool)
  }
  n165 = Enqueue Element(queue=w3, element="quit", error in (no error)=w5) -> (error out=w8:errorcluster)  [unwired: 1 in, 2 out]
  n166 = Close Reference(reference=w6, error in (no error)=w8) -> (error out=w2:errorcluster)
  n167 = for {
    N: 100 -> [_]
    tunnel: w4 -> [w267]
    shift-right: [w265] -> w13
    shift-left: w2 -> [w266]
    tunnel: [w262] -> w11
    stop <- w262 stop-if-true
    # "waits max 1 s to finish qeue"
    n168 = Get Queue Status(queue=w267, error in (no error)=w266) -> (error out=w265:errorcluster, # elements in queue=w263:i32)  [unwired: 1 in, 6 out]
    n169 = Wait (ms)(milliseconds to wait=u32 10) -> ()  [unwired: 1 out]
    n170 = Equal To 0?(x=w263) -> (x = 0?=w262:bool)
  }
  n171 = xnode "Error Ring"() -> ("error out"=w14:errorcluster)
  n172 = Not(x=w11) -> (.not. x?=w15:bool)
  n173 = call "Merge Error Ex.vi"("Is error? (False)"=w15, "main error in (no error)"=w13, "second error in"=w14) -> ("error out"=w12:errorcluster)  [unwired: 8 in]
  n174 = Release Queue(queue=w4, error in (no error)=w12) -> ()  [unwired: 1 in, 3 out]
